vi "PNA-X_GetFileInfo.vi"(0 "VISA IN":refnum<visa-resource-name>="TCPIP0::169.254.70.180::inst0::INSTR", 11 "error in":errorcluster, 12 "Path":string="D:\\State Files\\WAM_PRODUCTION.csa", 13 "Types":string(combo)="CSAR") -> (2 "file exists?(t)":bool=TRUE, 3 "files(ary)":string[](array[string])=["WAM_PRODUCTION.csa", "WAM_PRODUCTION_010423-1601 (2).csa", "WAM_PRODUCTION_010423-1601.csa", "WAM_PRODUCTION_012223-1129-BadReturnLoss.csa", "WAM_PRODUCTION_071222.csa"], 4 "VISA Out":refnum<visa-resource-name>="TCPIP0::169.254.70.180::inst0::INSTR", 15 "error out":errorcluster)   [LabVIEW 2018]
uses:
  PNA-X.lvlib
panel:
  out "Dir":string="D:\\State Files"
  out "name":string="WAM_PRODUCTION.csa"
  out "read":string="\"WAM_PRODUCTION.csa,WAM_PRODUCTION_010423-1601 (2).csa,WAM_PRODUCTION_010423-1601.csa,WAM_PRODUCTION_012223-1129-BadReturnLoss.csa,WAM_PRODUCTION_071222.csa\"\n"
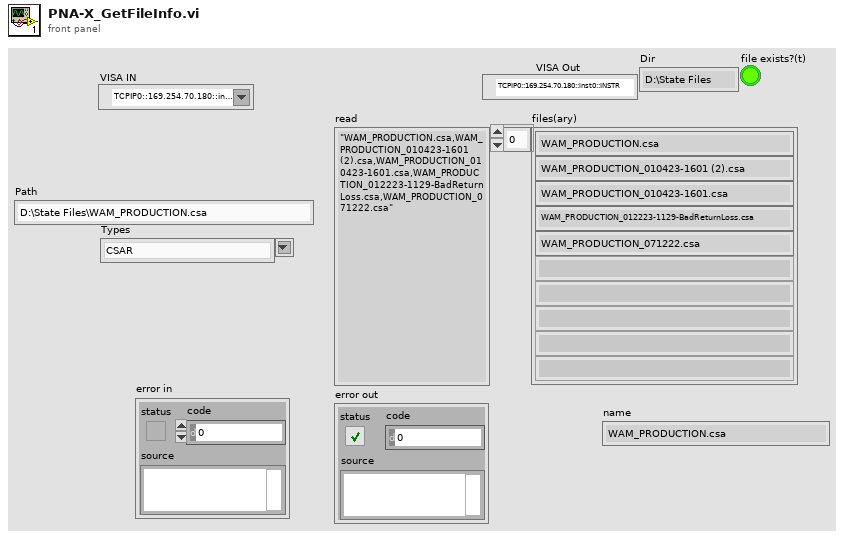
[diagram p1: front panel]
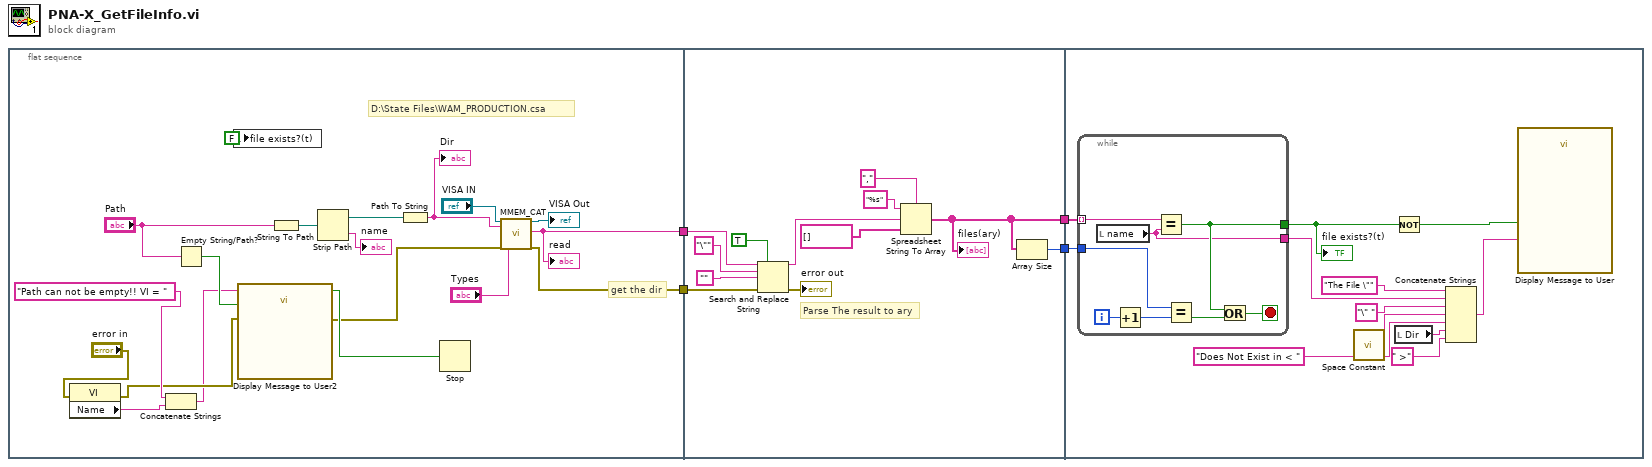
[diagram p0: block diagram]
diagram:
  n1 = flat-sequence {
    tunnel: [w23] -> w4
    tunnel: [w20] -> w3
    tunnel: w4 -> [w33]
    tunnel: w3 -> [w29]
    tunnel: [w25] -> w2
    tunnel: [w24] -> w1
    tunnel: w2 -> [w47]
    tunnel: w1 -> [w46]
    frame #0 {
      # "D:\\State Files\\WAM_PRODUCTION.csa"
      # "get the dir"
      n2 = property class="VI"(error in="error in") -> (error out=w6:errorcluster, "Name"=w8:string)  [unwired: 1 in, 1 out]
      n3 = Concatenate Strings("Path can not be empty!! VI = " ("Message"), w8) -> (w5:string)
      n4 = Empty String/Path?(string/path="Path") -> (empty?=w12:bool)
      n5 = local write "file exists?(t)"(FALSE ("x = y?")) -> ()
      n6 = call "Display Message to User2"("error in (no error)"=w6, "Enable"=w12, "Message"=w5) -> ("error out"=w10:errorcluster, "OK"=w11:bool)  [unwired: 7 in]
      n7 = String To Path(string="Path") -> (path=w16:path)
      n8 = Strip Path(path=w16) -> (stripped path=w18:path, name=→"name":string)
      n9 = Path To String(path=w18) -> (string=w17:string)
      "Dir" <- w17
      n10 = Stop(stop? (T)=w11) -> ()
      n11 = call "MMEM_CAT.vi"("VISA IN"="VISA IN", "Folder"=w17, "error in"=w10, "Types"="Types") -> ("VISA Out"=→"VISA Out":refnum<visa-resource-name>, "Data"=w23:string, "error out"=w20:errorcluster)  [unwired: 13 in]
      "read" <- w23
    }
    frame #1 {
      # "Parse The result to ary"
      n12 = Search and Replace String(replace all?=TRUE ("replace all? (F)"), input string=w33, search string="\"", replace string="", error in=w29) -> (result string=w34:string, error out=→"error out":errorcluster)  [unwired: 3 in, 2 out]
      n13 = Spreadsheet String To Array(delimiter (Tab)=",", format string="%s", spreadsheet string=w34, array type (2D Dbl)=string[] []) -> (array=w25:string[])
      "files(ary)" <- w25
      n14 = Array Size(array=w25) -> (size(s)=w24:i32)
    }
    frame #2 {
      n15 = while {
        tunnel: w47 -> [w55] mode=indexing
        tunnel: w46 -> [w54]
        tunnel: [w49] -> w45
        tunnel: [w48] -> w37
        i -> [w53]
        stop <- w50 stop-if-true
        n16 = local read "name"() -> (w48:string)
        n17 = Increment(x=w53) -> (x+1=w52:i32)
        n18 = Equal?(x=w55, y=w48) -> (x = y?=w49:bool)
        n19 = Equal?(x=w54, y=w52) -> (x = y?=w51:bool)
        n20 = Or(x=w49, y=w51) -> (x .or. y?=w50:bool)
      }
      "file exists?(t)" <- w45
      n21 = call <vilib>:"Space Constant.vi"() -> ("String"=w42:string)
      n22 = Not(x=w45) -> (.not. x?=w44:bool)
      n23 = local read "Dir"() -> (w40:string)
      n24 = Concatenate Strings("The File \"" ("string"), w37, "\" " ("string"), w42, "Does Not Exist in < " ("string"), w40, " >" ("string")) -> (w43:string)
      n25 = call "Display Message to User"("Enable"=w44, "Message"=w43) -> ()  [unwired: 8 in, 2 out]
    }
  }
